vi "AlliGator Add Action(s) to Stack.vi"   [LabVIEW 2021, in "AlliGator Action Engine.lvlib"]
doc: "Polymorphic VI with two versions:\n- AlliGator Add Action Array to Stack.vi\n- AlliGator Add Single Action to Stack.vi"
uses:
  AlliGator Action Engine.lvlib
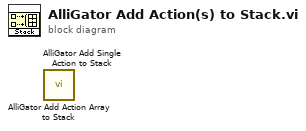
[diagram p0: block diagram]
diagram:
  n1 = call "AlliGator Add Action Array to Stack.vi"() -> ()  [unwired: 10 in, 2 out]
  n2 = call "AlliGator Add Single Action to Stack.vi"() -> ()  [unwired: 10 in, 2 out]
